vi "Build Unconfigured HTML.vi"(8 "error in (no error)":errorcluster, 11 "HomeHTTPController in":refnum<class "HomeHTTPController.lvclass">) -> (0 "error out":errorcluster, 2 "Unconfigured HTML":string="<html>\n    <head>\n        <title>Volatus</title>\n    </head>\n    <body>\n        <h1>Volatus</h1>\n        <p>The system is unconfigured. Upload a configuration below.</p>\n        <form name=\"new_config\" method=\"POST\" action=\"/config/new\" enctype=\"multipart/form-data\">\n            <p>System</p><input type=\"text\" name=\"system\"/>\n            <p>Cluster</p><input type=\"text\" name=\"cluster\"/>\n            <p>Node</p><input type=\"text\" name=\"node\"/>\n            <p>Config</p><input type=\"file\" name=\"config\" accept=\".vjson\"/>\n            <input type=\"submit\" value=\"submit\"/>\n        </form>\n    </body>\n</html>", 3 "HomeHTTPController out":refnum<class "HomeHTTPController.lvclass">)   [LabVIEW 2020, in "Volatus.lvlib" / "HomeHTTPController.lvclass"]
uses:
  HomeHTTPController.lvclass
  HomeHTTPController.lvclass/HomeHTTPController.ctl
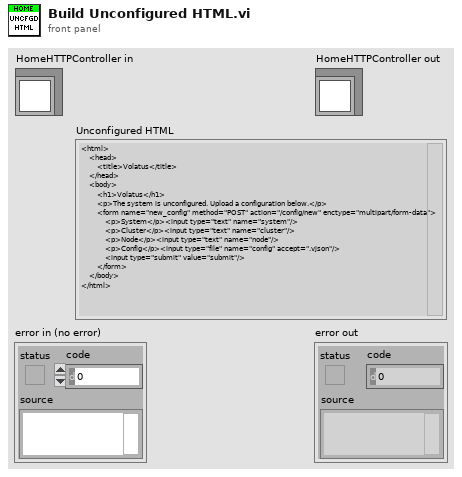
[diagram p1: front panel]
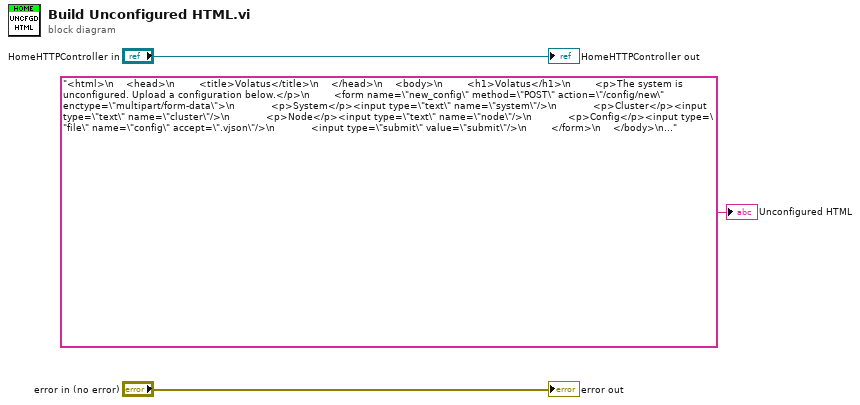
[diagram p0: block diagram]
diagram:
  "error out" <- "error in (no error)"
  "HomeHTTPController out" <- "HomeHTTPController in"
  "Unconfigured HTML" <- "<html>\n    <head>\n        <title>Volatus</title>\n    </head>\n    <body>\n        <h1>Volatus</h1>\n        <p>The system is unconfigured. Upload a configuration below.</p>\n        <form name=\"new_config\" method=\"POST\" action=\"/config/new\" enctype=\"multipart/form-data\">\n            <p>System</p><input type=\"text\" name=\"system\"/>\n            <p>Cluster</p><input type=\"text\" name=\"cluster\"/>\n            <p>Node</p><input type=\"text\" name=\"node\"/>\n            <p>Config</p><input type=\"file\" name=\"config\" accept=\".vjson\"/>\n            <input type=\"submit\" value=\"submit\"/>\n        </form>\n    </body>\n</html>"
